vi "Requests.vi"(8 "error in (no error)":errorcluster, 9 "write enable":bool=TRUE, 11 "ICPCON ET7024 in":refnum<class "ICPCON ET-7024.lvclass">) -> (0 "error out":errorcluster, 3 "ICPCON ET7024 out":refnum<class "ICPCON ET-7024.lvclass">)   [LabVIEW 2021, in "ICPCON ET-7024.lvclass"]
uses:
  ICPCON ET-7024.lvclass
  D:/my_projects/projects/21/Master CR/Master CR.lvclass
  D:/my_projects/projects/21/Master CR/Devices/ET7000/TCP/TCP.lvclass
  Master CR.lvclass/Master CR.ctl
  Modbus_v121c/Modbus Data Unit/Modbus Data Unit.lvclass/Modbus Data Unit.ctl
  Modbus_v121c/Network Protocol/Network Master/Network Master.lvclass/Network Master.ctl
  Modbus_v121c/Master Function Definition/Read Discrete Inputs Request.vi
  Modbus_v121c/Network Protocol/Network Master/Read write Master.vi
  Modbus_v121c/Master Function Definition/Read Discrete Inputs Response.vi
  Network Protocol/Read Network Protocol.vi
  Modbus_v121c/Modbus Data Unit/Construct PDU.vi
  Modbus_v121c/Utility/Bytes to Bits.vi
  Modbus_v121c/Master Function Definition/Function code mismatch error.vi
  Modbus_v121c/Data Model/Error Generator.vi
  Modbus_v121c/Modbus Data Unit/Deconstruct PDU.vi
  TCP/TCP.lvclass
  Modbus_v121c/Network Protocol/Network Master/Network Master.lvclass
  Modbus_v121c/Modbus Data Unit/Modbus Data Unit.lvclass
  Modbus_v121c/Data Model/Device Data Model.lvclass
  Modbus_v121c/Transmission Data Unit/Transmission Data Unit.lvclass
  Master CR.lvclass
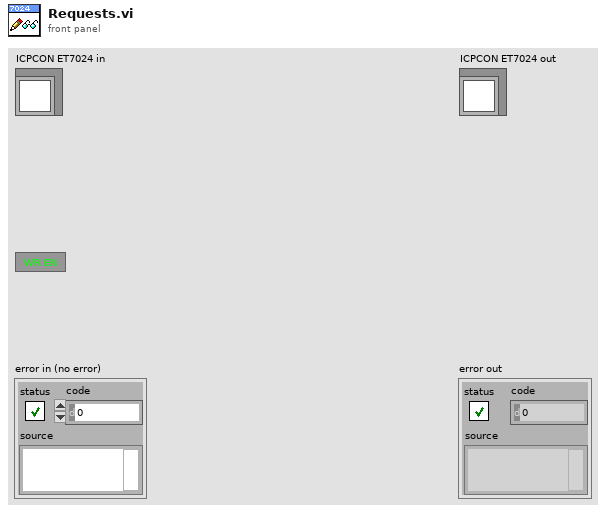
[diagram p1: front panel]
types:
  T1 = typedef "Device Data Model.lvclass/N channel.ctl" = cluster{"N DI channel":i32, "N DO channel":i32, "N AI channel":i32, "N AO channel":i32}
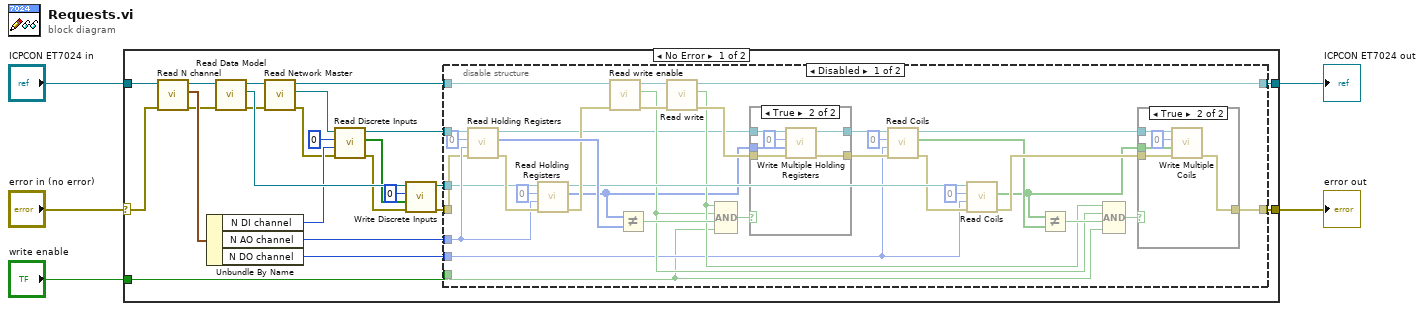
[diagram p0: block diagram]
diagram:
  n1 = case shown="No Error" "error in (no error)" {
    selector: "error in (no error)" -> [w26 w82]
    tunnel: [w12 w82] -> w3
    tunnel: [w11 w81] -> w4
    tunnel: "ICPCON ET7024 in" -> [w28 w81]
    tunnel: "write enable" -> [w13 _]
    frame No Error {
      n2 = call "Read N channel.vi"("error in (no error)"=w26, "Master CR in"=w28) -> ("error out"=w25:errorcluster, "N channel"=w29:T1, "Master CR out"=w27:refnum<class "ICPCON ET-7024.lvclass">)  [unwired: 7 in]
      n3 = Unbundle By Name(w29) -> ("N DI channel"=w19:i32, "N AO channel"=w24:i32, "N DO channel"=w14:i32)
      n4 = call "Read Data Model.vi"("error in (no error)"=w25, "Master CR in"=w27) -> ("error out"=w9:errorcluster, "Data Model"=w23:refnum<class "Device Data Model.lvclass">, "Master CR out"=w10:refnum<class "ICPCON ET-7024.lvclass">)  [unwired: 7 in]
      n5 = call "Read Network Master.vi"("error in (no error)"=w9, "TCP in"=w10) -> ("error out"=w8:errorcluster, "Network Master"=w7:refnum<class "Network Master.lvclass">, "TCP out"=w6:refnum<class "ICPCON ET-7024.lvclass">)  [unwired: 7 in]
      n6 = call "Read Discrete Inputs.vi"("error in (no error)"=w8, "number of discrete inputs"=w19, "starting address"=u16 0, "Modbus master in"=w7) -> ("error out"=w17:errorcluster, "discrete input values"=w18:bool[], "Modbus master out"=w16:refnum<class "Network Master.lvclass">)  [unwired: 5 in]
      n7 = call-dynamic "Write Discrete Inputs.vi"("error in (no error)"=w17, "input values"=w18, "starting address"=u16 0, "Device Data Model in"=w23) -> ("error out"=w15:errorcluster, "Device Data Model out"=w22:refnum<class "Device Data Model.lvclass">)  [unwired: 6 in]
      n8 = disable-structure shown="Disabled" {
        disable-tunnel: w24 -> [w54 _]
        disable-tunnel: w22 -> [w53 _]
        disable-tunnel: w16 -> [w52 _]
        disable-tunnel: w15 -> [w51 w79]
        disable-tunnel: w14 -> [w38 _]
        disable-tunnel: w13 -> [w36 _]
        disable-tunnel: [w35 w79] -> w12
        disable-tunnel: [w32 w80] -> w11
        disable-tunnel: w6 -> [w30 w80]
        frame Disabled {
          n9 = call "Read Holding Registers.vi"("error in (no error)"=w51, "number of holding registers"=w54, "starting address"=u16 0, "Modbus master in"=w52) -> ("error out"=w55:errorcluster, "register values"=w57:u16[], "Modbus master out"=w31:refnum<class "Network Master.lvclass">)  [unwired: 5 in]
          n10 = call-dynamic "Read Holding Registers.vi"("error in"=w55, "number of registers"=w54, "starting address"=u16 0, "device data model in"=w53) -> ("error out"=w56:errorcluster, "data"=w34:u16[], "device data model out"=w48:refnum<class "Device Data Model.lvclass">)  [unwired: 5 in]
          n11 = call "Read write enable.vi"("error in (no error)"=w56, "Master CR in"=w30) -> ("error out"=w61:errorcluster, "write enable"=w45:bool, "Master CR out"=w62:refnum<class "ICPCON ET-7024.lvclass">)  [unwired: 7 in]
          n12 = Not Equal?(x=w34, y=w57) -> (x != y?=w63:bool)
          n13 = call "Read write.vi"("error in (no error)"=w61, "Master CR in"=w62) -> ("error out"=w60:errorcluster, "Write"=w46:bool, "Master CR out"=w32:refnum<class "ICPCON ET-7024.lvclass">)  [unwired: 7 in]
          n14 = Compound Arithmetic op=AND(w46, w45, w63, w36) -> (w64:bool)
          n15 = case shown="True" w64 {
            tunnel: w60 -> [w66 w71]
            tunnel: [w66 w69] -> w39
            tunnel: w34 -> [_ w70]
            tunnel: [w65 w68] -> w40
            tunnel: w31 -> [w65 w67]
            frame False {
            }
            frame True {
              n16 = call "Write Multiple Holding Registers.vi"("error in (no error)"=w71, "holding register values"=w70, "starting address"=u16 0, "Modbus master in"=w67) -> ("error out"=w69:errorcluster, "Modbus master out"=w68:refnum<class "Network Master.lvclass">)  [unwired: 6 in]
            }
          }
          n17 = call "Read Coils.vi"("error in (no error)"=w39, "number of coils"=w38, "starting address"=u16 0, "Modbus master in"=w40) -> ("error out"=w42:errorcluster, "coil values"=w43:bool[], "Modbus master out"=w44:refnum<class "Network Master.lvclass">)  [unwired: 5 in]
          n18 = call-dynamic "Read Coils.vi"("error in"=w42, "number of coils"=w38, "starting address"=u16 0, "device data model in"=w48) -> ("error out"=w47:errorcluster, "data"=w33:bool[])  [unwired: 5 in, 1 out]
          n19 = Not Equal?(x=w33, y=w43) -> (x != y?=w50:bool)
          n20 = Compound Arithmetic op=AND(w46, w45, w50, w36) -> (w49:bool)
          n21 = case shown="True" w49 {
            tunnel: w47 -> [w73 w77]
            tunnel: [w73 w74] -> w35
            tunnel: w33 -> [_ w76]
            tunnel: w44 -> [_ w78]
            frame False {
            }
            frame True {
              n22 = call "Write Multiple Coils.vi"("error in (no error)"=w77, "coil values"=w76, "starting address"=u16 0, "Modbus master in"=w78) -> ("error out"=w74:errorcluster)  [unwired: 6 in, 1 out]
            }
          }
        }
        frame Enabled {
        }
      }
    }
    frame Error {
    }
  }
  "error out" <- w3
  "ICPCON ET7024 out" <- w4
